vi "main.vi"() -> ()   [LabVIEW 2018]
uses:
  AutoExp/AutoExp.lvclass
  AutoExp/AutoExp.lvclass/AutoExp.ctl
  Channel/Channel.lvclass/Channel.ctl
  File interpreter/File interpreter.lvclass/File interpreter.ctl
  Channel/Channel.lvclass
  RxTx/RxTx.lvclass
  State Machine/State Machine.lvclass
  File interpreter/File interpreter.lvclass
  JSON reader/JSON reader.lvclass
  Interface/Interface.lvclass
panel:
  out "Error Out":errorcluster
  in  "Tab Control":enum32{"Acquisition", "JSON Tool"}(tab)
  out "Wait time":u16
  out "Wait time":u16
  out "Wait time":u16
  out "Wait time":u16
  out "Serial Number":u16
  out "Channel 4":bool
  out "CH4 Acquiring":bool
  out "Exp Time":dbl
  out "Temperature":i16
  out "CH4 CCD Status":string
  out "CH4 Exposures done":u8(slide) caption="Exposures done" max=1 scale=0.0..1.0
  out "CH4 Image Name":string
  out "CH4 Temp Status":string
  out "Serial Number":u16
  out "Channel 3":bool
  out "CH3 Acquiring":bool
  out "Exp Time":dbl
  out "Temperature":i16
  out "CH3 CCD Status":string
  out "CH3 Exposures done":u8(slide) caption="Exposures done" max=1 scale=0.0..1.0
  out "CH3 Image Name":string
  out "CH3 Temp Status":string
  out "Serial Number":u16
  out "Channel 2":bool
  out "CH2 Acquiring":bool
  out "Exp Time":dbl
  out "Temperature":i16
  out "CH2 CCD Status":string
  out "CH2 Exposures done":u8(slide) caption="Exposures done" max=1 scale=0.0..1.0
  out "CH2 Image Name":string
  out "CH2 Temp Status":string
  in  "Stop Application":bool
  out "Serial Number":u16
  out "Channel 1":bool
  in  "Start Acquisition":bool
  out "Acquiring":bool
  in  "Script file":path
  out "Exp Time":dbl
  out "Temperature":i16
  out "CCD Status":string
  out "Exposures done":u8(slide) max=1 scale=0.0..10.0
  out "Image Name":string
  out "Temp Status":string
  in  "Create JSON string":bool
  out "JSON string":string
  in  "AutoExp.lvclass":refnum<class "AutoExp.lvclass">
  # "Welcome to the SPARC4 Automatic Experiments Interface (AutoExp)"
  # "Channel 1"
  # "Channel 2"
  # "Channel 3"
  # "Channel 4"
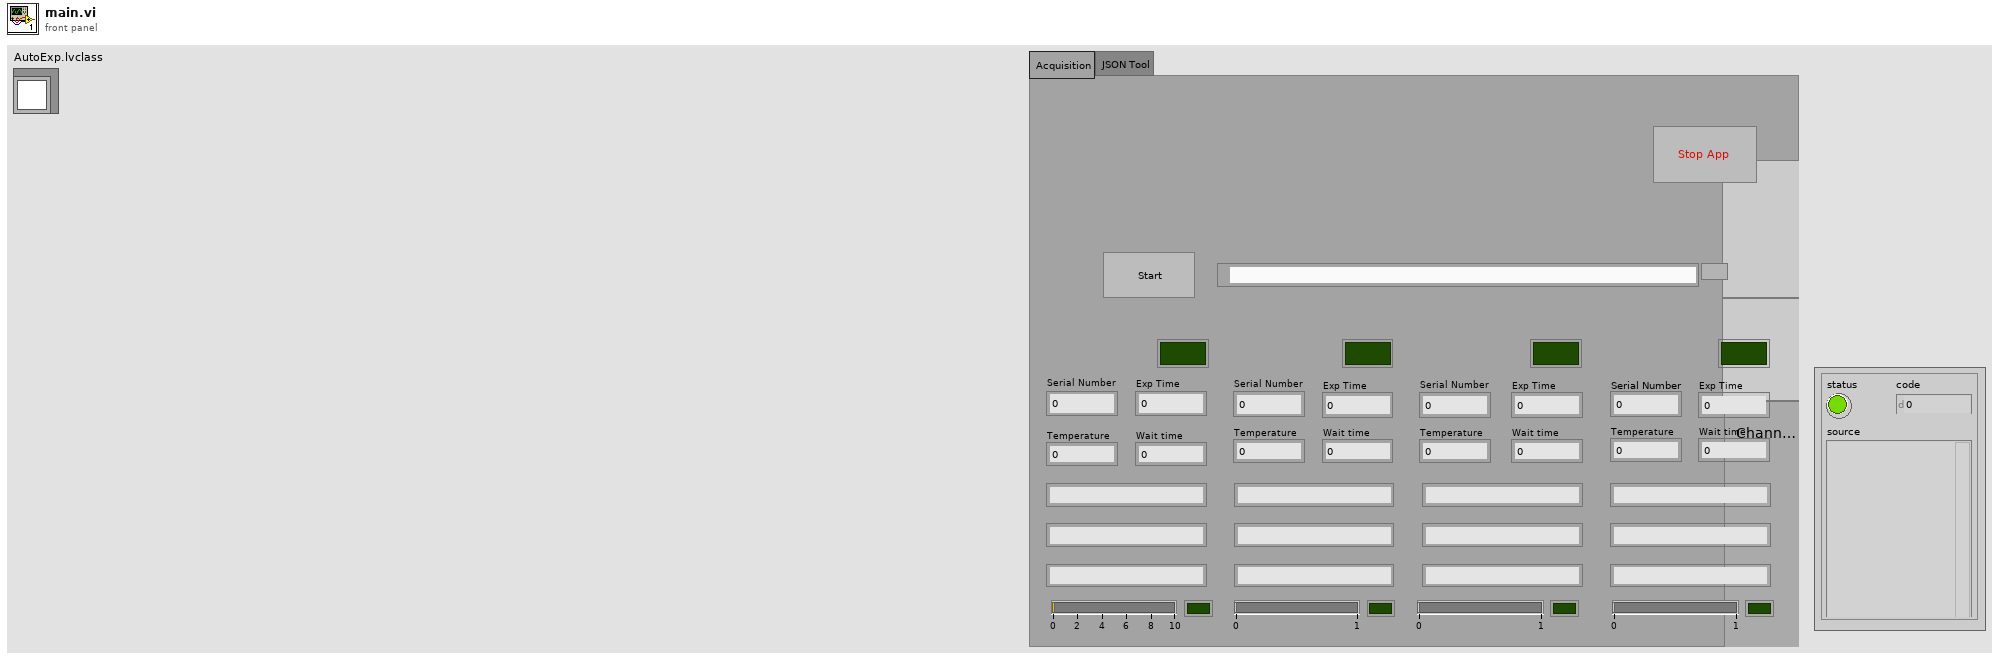
[diagram p1: front panel]
types:
  T1 = cluster{"CUBE_EXPOSURE_TIME":sgl, "CUBES_DONE":u16, "LAST_IMAGE_NAME":string, "DISK_SPACE":u16, "FRAMES_DONE":u16, "CCD_STATUS":string, "CURRENT_TEMPERATURE":i16, "TEMPERATURE_STATUS":string, "FRAME_EXPOSURE_TIME":u16, "CCD_ON_OFF":bool, "SERIAL_NUMBER":u16, "ACQUIRING":bool}
  T2 = cluster{"Exposure Time":sgl, "Pre-amp gain":u8, "Readout Rate":u8, "EM Mode":u8, "EM Gain":u16, "Binning":u16, "Initial Line":u16, "Initial Cloumn":u16, "Final Line":u16, "Final Column":u16, "Kinetic Series Length":u32, "Shutter Mode":u8, "Cooler ON/OFF":u16, "Temperature":i8, "Cubes":u32, "Trigger":u16, "Set Trigger":bool}
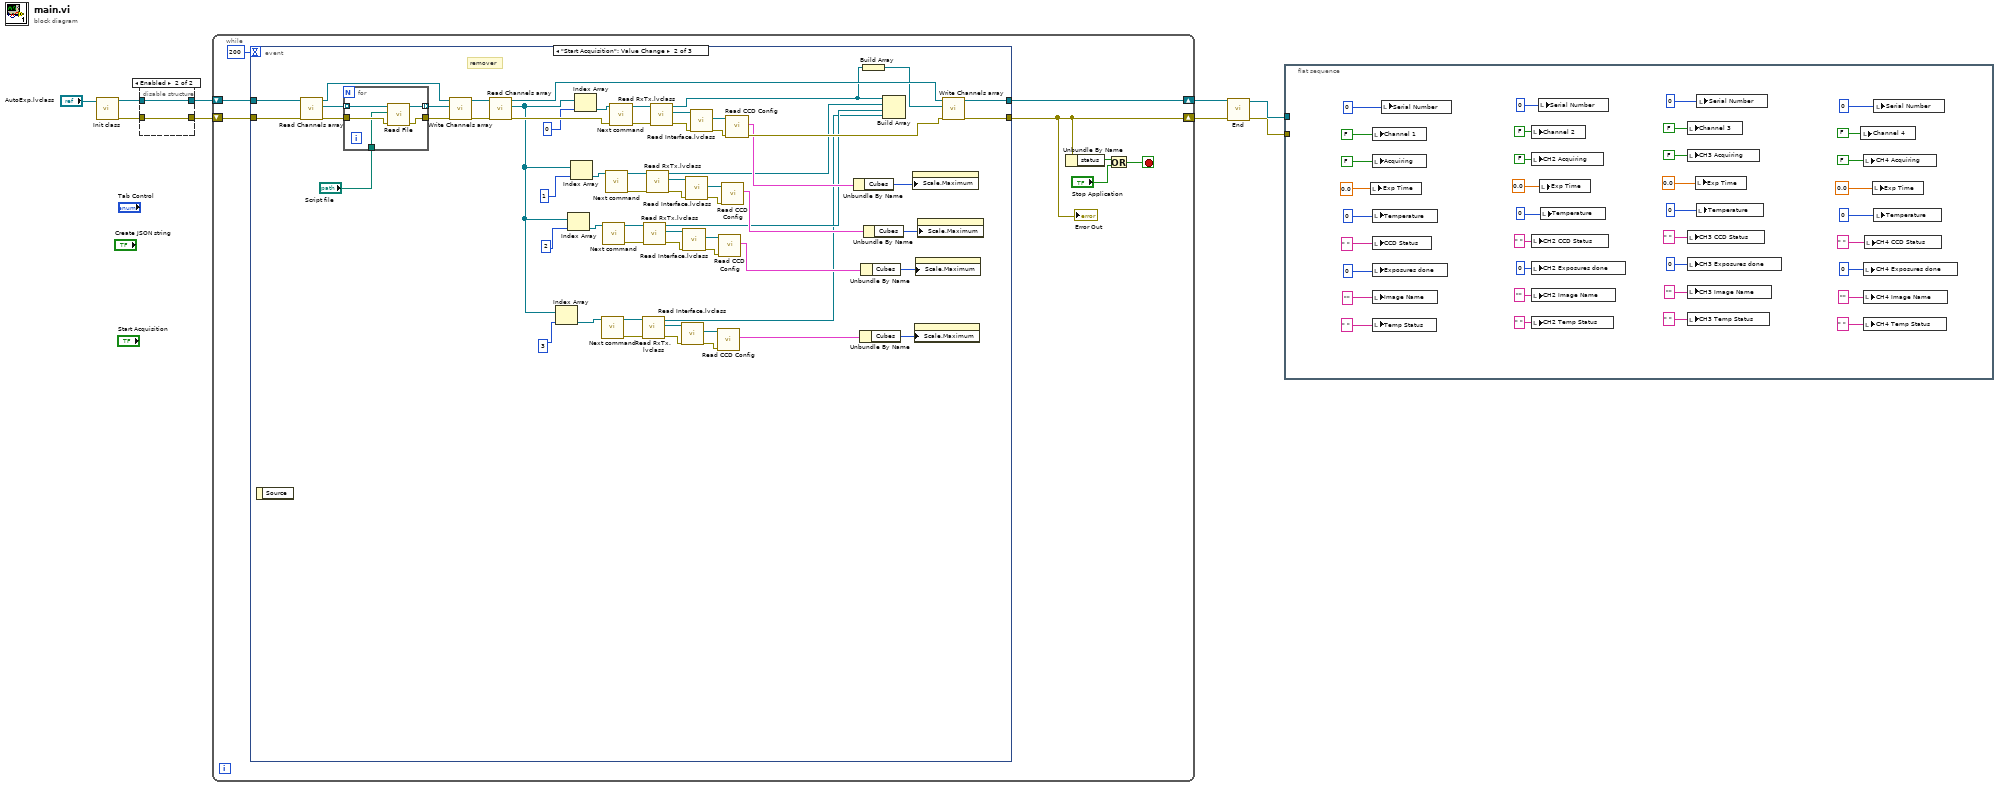
[diagram p0: block diagram]
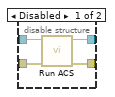
[diagram p2: hidden frame]
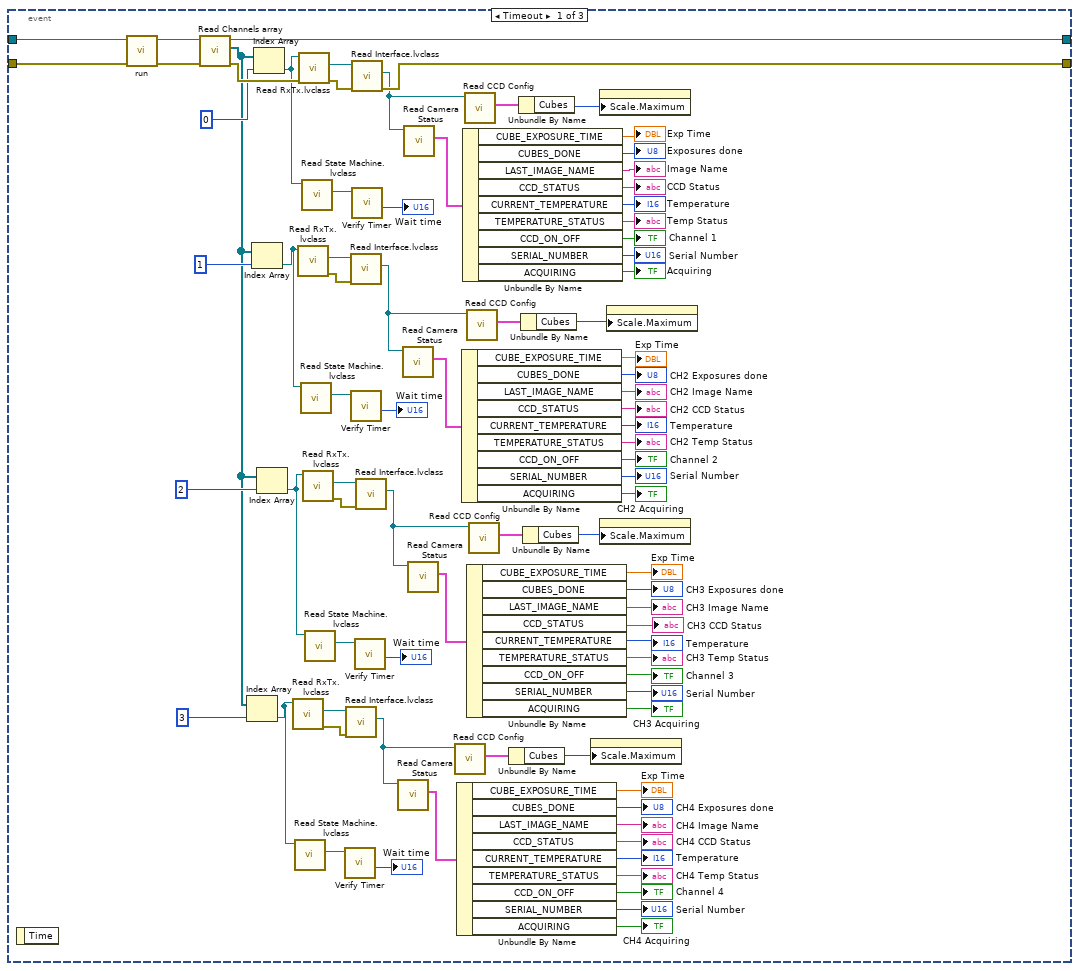
[diagram p3: hidden frame]
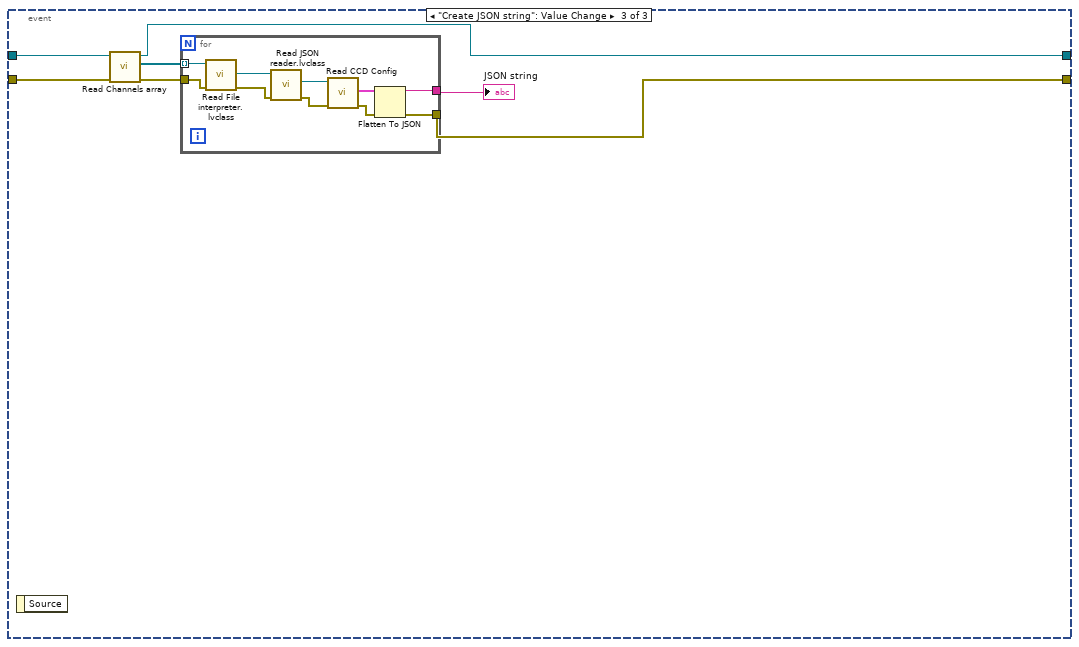
[diagram p4: hidden frame]
diagram:
  n1 = call "Init class.vi"("AutoExp in"="AutoExp.lvclass") -> ("error out"=w4:errorcluster, "AutoExp out"=w7:refnum<class "AutoExp.lvclass">)  [unwired: 9 in]
  n2 = disable-structure shown="Enabled" {
    disable-tunnel: w7 -> [w13 w15]
    disable-tunnel: [w12 w15] -> w6
    disable-tunnel: [w11 w14] -> w5
    disable-tunnel: w4 -> [w10 w14]
    frame Disabled {
      n3 = call "Run ACS.vi"("error in (no error)"=w10, "AutoExp in"=w13) -> ("error out"=w11:errorcluster, "AutoExp out"=w12:refnum<class "AutoExp.lvclass">)  [unwired: 8 in]
    }
    frame Enabled {
    }
  }
  n4 = while {
    shift-right: [w16] -> w1
    shift-left: w5 -> [w20]
    shift-right: [w21] -> w9
    shift-left: w6 -> [w22]
    stop <- w19 stop-if-true
    n5 = event shown="[1] \"Start Acquisition\": Value Change" {
      selector: _ -> [_ _ _]
      dyn-events: _ -> [_ _ _]
      timeout: 200 -> [_ _ _]
      tunnel: w22 -> [w107 w115 w180]
      tunnel: [w102 w168 w175] -> w21
      tunnel: [w101 w167 w174] -> w16
      tunnel: w20 -> [w106 w114 w179]
      event Timeout {
        n6 = event-data() -> ()  [unwired: 1 in, 1 out]
        n7 = call "run.vi"("error in (no error)"=w106, "AutoExp in"=w107) -> ("error out"=w104:errorcluster, "AutoExp out"=w105:refnum<class "AutoExp.lvclass">)  [unwired: 8 in]
        n8 = call "Read Channels array.vi"("error in (no error)"=w104, "AutoExp in"=w105) -> ("error out"=w103:errorcluster, "Channels array"=w65:refnum<class "Channel.lvclass">[], "AutoExp out"=w102:refnum<class "AutoExp.lvclass">)  [unwired: 7 in]
        n9 = Index Array(array=w65, index=3) -> (element=w41:refnum<class "Channel.lvclass">)
        n10 = Index Array(array=w65, index=1) -> (element=w47:refnum<class "Channel.lvclass">)
        n11 = Index Array(array=w65, index=0) -> (element=w51:refnum<class "Channel.lvclass">)
        n12 = Index Array(array=w65, index=2) -> (element=w44:refnum<class "Channel.lvclass">)
        n13 = call "Read RxTx.lvclass.vi"("Channel in"=w41) -> ("error out"=w63:errorcluster, "RxTx.lvclass"=w64:refnum<class "RxTx.lvclass">)  [unwired: 8 in, 1 out]
        n14 = call "Read State Machine.lvclass.vi"("Channel in"=w41) -> ("State Machine.lvclass"=w42:refnum<class "State Machine.lvclass">)  [unwired: 8 in, 2 out]
        n15 = call "Read RxTx.lvclass.vi"("Channel in"=w47) -> ("error out"=w88:errorcluster, "RxTx.lvclass"=w87:refnum<class "RxTx.lvclass">)  [unwired: 8 in, 1 out]
        n16 = call "Read RxTx.lvclass.vi"("error in (no error)"=w103, "Channel in"=w51) -> ("error out"=w99:errorcluster, "RxTx.lvclass"=w100:refnum<class "RxTx.lvclass">)  [unwired: 7 in, 1 out]
        n17 = call "Read State Machine.lvclass.vi"("Channel in"=w47) -> ("State Machine.lvclass"=w48:refnum<class "State Machine.lvclass">)  [unwired: 8 in, 2 out]
        n18 = call "Read State Machine.lvclass.vi"("Channel in"=w51) -> ("State Machine.lvclass"=w50:refnum<class "State Machine.lvclass">)  [unwired: 8 in, 2 out]
        n19 = call "Read RxTx.lvclass.vi"("Channel in"=w44) -> ("error out"=w74:errorcluster, "RxTx.lvclass"=w75:refnum<class "RxTx.lvclass">)  [unwired: 8 in, 1 out]
        n20 = call "Read State Machine.lvclass.vi"("Channel in"=w44) -> ("State Machine.lvclass"=w45:refnum<class "State Machine.lvclass">)  [unwired: 8 in, 2 out]
        n21 = call "Verify Timer.vi"("State Machine in"=w42) -> ("elapsed time"=→"Wait time":u16)  [unwired: 7 in, 3 out]
        n22 = call "Read Interface.lvclass.vi"("error in (no error)"=w63, "RxTx in"=w64) -> ("Interface.lvclass"=w25:refnum<class "Interface.lvclass">)  [unwired: 7 in, 2 out]
        n23 = call "Read Interface.lvclass.vi"("error in (no error)"=w88, "RxTx in"=w87) -> ("Interface.lvclass"=w31:refnum<class "Interface.lvclass">)  [unwired: 7 in, 2 out]
        n24 = call "Verify Timer.vi"("State Machine in"=w48) -> ("elapsed time"=→"Wait time":u16)  [unwired: 7 in, 3 out]
        n25 = call "Read Interface.lvclass.vi"("error in (no error)"=w99, "RxTx in"=w100) -> ("error out"=w101:errorcluster, "Interface.lvclass"=w35:refnum<class "Interface.lvclass">)  [unwired: 7 in, 1 out]
        n26 = call "Verify Timer.vi"("State Machine in"=w50) -> ("elapsed time"=→"Wait time":u16)  [unwired: 7 in, 3 out]
        n27 = call "Verify Timer.vi"("State Machine in"=w45) -> ("elapsed time"=→"Wait time":u16)  [unwired: 7 in, 3 out]
        n28 = call "Read Interface.lvclass.vi"("error in (no error)"=w74, "RxTx in"=w75) -> ("Interface.lvclass"=w28:refnum<class "Interface.lvclass">)  [unwired: 7 in, 2 out]
        n29 = call "Read Camera Status.vi"("Interface in"=w25) -> ("Camera Status"=w57:T1)  [unwired: 8 in, 2 out]
        n30 = call "Read Camera Status.vi"("Interface in"=w31) -> ("Camera Status"=w89:T1)  [unwired: 8 in, 2 out]
        n31 = call "Read Camera Status.vi"("Interface in"=w35) -> ("Camera Status"=w98:T1)  [unwired: 8 in, 2 out]
        n32 = call "Read Camera Status.vi"("Interface in"=w28) -> ("Camera Status"=w73:T1)  [unwired: 8 in, 2 out]
        n33 = call "Read CCD Config.vi"("Interface in"=w25) -> ("CCD Config"=w26:T2)  [unwired: 8 in, 2 out]
        n34 = Unbundle By Name(w57) -> ("CUBE_EXPOSURE_TIME"=→"Exp Time":sgl, "CUBES_DONE"=→"CH4 Exposures done":u16, "LAST_IMAGE_NAME"=→"CH4 Image Name":string, "CCD_STATUS"=→"CH4 CCD Status":string, "CURRENT_TEMPERATURE"=→"Temperature":i16, "TEMPERATURE_STATUS"=→"CH4 Temp Status":string, "CCD_ON_OFF"=→"Channel 4":bool, "SERIAL_NUMBER"=→"Serial Number":u16, "ACQUIRING"=→"CH4 Acquiring":bool)
        n35 = Unbundle By Name(w89) -> ("CUBE_EXPOSURE_TIME"=→"Exp Time":sgl, "CUBES_DONE"=→"CH2 Exposures done":u16, "LAST_IMAGE_NAME"=→"CH2 Image Name":string, "CCD_STATUS"=→"CH2 CCD Status":string, "CURRENT_TEMPERATURE"=→"Temperature":i16, "TEMPERATURE_STATUS"=→"CH2 Temp Status":string, "CCD_ON_OFF"=→"Channel 2":bool, "SERIAL_NUMBER"=→"Serial Number":u16, "ACQUIRING"=→"CH2 Acquiring":bool)
        n36 = Unbundle By Name(w98) -> ("CUBE_EXPOSURE_TIME"=→"Exp Time":sgl, "CUBES_DONE"=→"Exposures done":u16, "LAST_IMAGE_NAME"=→"Image Name":string, "CCD_STATUS"=→"CCD Status":string, "CURRENT_TEMPERATURE"=→"Temperature":i16, "TEMPERATURE_STATUS"=→"Temp Status":string, "CCD_ON_OFF"=→"Channel 1":bool, "SERIAL_NUMBER"=→"Serial Number":u16, "ACQUIRING"=→"Acquiring":bool)
        n37 = call "Read CCD Config.vi"("Interface in"=w35) -> ("CCD Config"=w34:T2)  [unwired: 8 in, 2 out]
        n38 = call "Read CCD Config.vi"("Interface in"=w31) -> ("CCD Config"=w32:T2)  [unwired: 8 in, 2 out]
        n39 = Unbundle By Name(w73) -> ("CUBE_EXPOSURE_TIME"=→"Exp Time":sgl, "CUBES_DONE"=→"CH3 Exposures done":u16, "LAST_IMAGE_NAME"=→"CH3 Image Name":string, "CCD_STATUS"=→"CH3 CCD Status":string, "CURRENT_TEMPERATURE"=→"Temperature":i16, "TEMPERATURE_STATUS"=→"CH3 Temp Status":string, "CCD_ON_OFF"=→"Channel 3":bool, "SERIAL_NUMBER"=→"Serial Number":u16, "ACQUIRING"=→"CH3 Acquiring":bool)
        n40 = call "Read CCD Config.vi"("Interface in"=w28) -> ("CCD Config"=w29:T2)  [unwired: 8 in, 2 out]
        n41 = Unbundle By Name(w26) -> ("Cubes"=w24:u32)
        n42 = Unbundle By Name(w34) -> ("Cubes"=w33:u32)
        n43 = Unbundle By Name(w32) -> ("Cubes"=w30:u32)
        n44 = Unbundle By Name(w29) -> ("Cubes"=w27:u32)
        n45 = property on="CH4 Exposures done" class="Slide (strict)"("Scale.Maximum"=w24) -> ()  [unwired: 2 in, 2 out]
        n46 = property on="Exposures done" class="Slide (strict)"("Scale.Maximum"=w33) -> ()  [unwired: 2 in, 2 out]
        n47 = property on="CH3 Exposures done" class="Slide (strict)"("Scale.Maximum"=w27) -> ()  [unwired: 2 in, 2 out]
        n48 = property on="CH2 Exposures done" class="Slide (strict)"("Scale.Maximum"=w30) -> ()  [unwired: 2 in, 2 out]
      }
      event "Start Acquisition": Value Change {
        # "remover"
        n49 = event-data() -> ()  [unwired: 1 in, 1 out]
        n50 = call "Read Channels array.vi"("error in (no error)"=w114, "AutoExp in"=w115) -> ("error out"=w118:errorcluster, "Channels array"=w120:refnum<class "Channel.lvclass">[], "AutoExp out"=w116:refnum<class "AutoExp.lvclass">)  [unwired: 7 in]
        n51 = for {
          tunnel: w120 -> [w173] mode=indexing
          tunnel: [w172] -> w119 mode=indexing
          tunnel: w118 -> [w171]
          tunnel: [w170] -> w117
          tunnel: "Script file" -> [w169]
          n52 = call "Read File.vi"("error in (no error)"=w171, "file path (use dialog)"=w169, "Channel in"=w173) -> ("error out"=w170:errorcluster, "Channel out"=w172:refnum<class "Channel.lvclass">)  [unwired: 7 in]
        }
        n53 = call "Write Channels array.vi"("error in (no error)"=w117, "Channels array"=w119, "AutoExp in"=w116) -> ("error out"=w112:errorcluster, "AutoExp out"=w113:refnum<class "AutoExp.lvclass">)  [unwired: 7 in]
        n54 = call "Read Channels array.vi"("error in (no error)"=w112, "AutoExp in"=w113) -> ("error out"=w165:errorcluster, "Channels array"=w110:refnum<class "Channel.lvclass">[], "AutoExp out"=w166:refnum<class "AutoExp.lvclass">)  [unwired: 7 in]
        n55 = Index Array(array=w110, index=3) -> (element=w131:refnum<class "Channel.lvclass">)
        n56 = Index Array(array=w110, index=2) -> (element=w142:refnum<class "Channel.lvclass">)
        n57 = Index Array(array=w110, index=1) -> (element=w148:refnum<class "Channel.lvclass">)
        n58 = Index Array(array=w110, index=0) -> (element=w156:refnum<class "Channel.lvclass">)
        n59 = call "Next command.vi"("Channel in"=w131) -> ("error out"=w133:errorcluster, "Channel out"=w130:refnum<class "Channel.lvclass">)  [unwired: 9 in]
        n60 = call "Next command.vi"("Channel in"=w142) -> ("error out"=w140:errorcluster, "Channel out"=w143:refnum<class "Channel.lvclass">)  [unwired: 9 in]
        n61 = call "Next command.vi"("Channel in"=w148) -> ("error out"=w150:errorcluster, "Channel out"=w147:refnum<class "Channel.lvclass">)  [unwired: 9 in]
        n62 = call "Next command.vi"("error in (no error)"=w165, "Channel in"=w156) -> ("error out"=w162:errorcluster, "Channel out"=w163:refnum<class "Channel.lvclass">)  [unwired: 8 in]
        n63 = call "Read RxTx.lvclass.vi"("error in (no error)"=w133, "Channel in"=w130) -> ("error out"=w134:errorcluster, "RxTx.lvclass"=w129:refnum<class "RxTx.lvclass">, "Channel out"=w122:refnum<class "Channel.lvclass">)  [unwired: 7 in]
        n64 = call "Read RxTx.lvclass.vi"("error in (no error)"=w140, "Channel in"=w143) -> ("error out"=w139:errorcluster, "RxTx.lvclass"=w144:refnum<class "RxTx.lvclass">, "Channel out"=w123:refnum<class "Channel.lvclass">)  [unwired: 7 in]
        n65 = call "Read RxTx.lvclass.vi"("error in (no error)"=w150, "Channel in"=w147) -> ("error out"=w151:errorcluster, "RxTx.lvclass"=w146:refnum<class "RxTx.lvclass">, "Channel out"=w124:refnum<class "Channel.lvclass">)  [unwired: 7 in]
        n66 = call "Read RxTx.lvclass.vi"("error in (no error)"=w162, "Channel in"=w163) -> ("error out"=w160:errorcluster, "RxTx.lvclass"=w161:refnum<class "RxTx.lvclass">, "Channel out"=w109:refnum<class "Channel.lvclass">)  [unwired: 7 in]
        n67 = call "Read Interface.lvclass.vi"("error in (no error)"=w134, "RxTx in"=w129) -> ("error out"=w136:errorcluster, "Interface.lvclass"=w135:refnum<class "Interface.lvclass">)  [unwired: 7 in, 1 out]
        n68 = call "Read Interface.lvclass.vi"("error in (no error)"=w139, "RxTx in"=w144) -> ("error out"=w137:errorcluster, "Interface.lvclass"=w138:refnum<class "Interface.lvclass">)  [unwired: 7 in, 1 out]
        n69 = call "Read Interface.lvclass.vi"("error in (no error)"=w151, "RxTx in"=w146) -> ("error out"=w153:errorcluster, "Interface.lvclass"=w152:refnum<class "Interface.lvclass">)  [unwired: 7 in, 1 out]
        n70 = call "Read Interface.lvclass.vi"("error in (no error)"=w160, "RxTx in"=w161) -> ("error out"=w158:errorcluster, "Interface.lvclass"=w159:refnum<class "Interface.lvclass">)  [unwired: 7 in, 1 out]
        n71 = call "Read CCD Config.vi"("error in (no error)"=w136, "Interface in"=w135) -> ("CCD Config"=w128:T2)  [unwired: 7 in, 2 out]
        n72 = call "Read CCD Config.vi"("error in (no error)"=w137, "Interface in"=w138) -> ("CCD Config"=w126:T2)  [unwired: 7 in, 2 out]
        n73 = call "Read CCD Config.vi"("error in (no error)"=w153, "Interface in"=w152) -> ("CCD Config"=w154:T2)  [unwired: 7 in, 2 out]
        n74 = call "Read CCD Config.vi"("error in (no error)"=w158, "Interface in"=w159) -> ("error out"=w164:errorcluster, "CCD Config"=w157:T2)  [unwired: 7 in, 1 out]
        n75 = Unbundle By Name(w157) -> ("Cubes"=w111:u32)
        n76 = Unbundle By Name(w128) -> ("Cubes"=w127:u32)
        n77 = Unbundle By Name(w126) -> ("Cubes"=w125:u32)
        n78 = Build Array(w109) -> (w108:refnum<class "Channel.lvclass">[])
        n79 = Unbundle By Name(w154) -> ("Cubes"=w145:u32)
        n80 = Build Array(w109, w124, w123, w122) -> ()  [unwired: 1 out]
        n81 = property on="Exposures done" class="Slide (strict)"("Scale.Maximum"=w111) -> ()  [unwired: 2 in, 2 out]
        n82 = property on="CH4 Exposures done" class="Slide (strict)"("Scale.Maximum"=w127) -> ()  [unwired: 2 in, 2 out]
        n83 = property on="CH3 Exposures done" class="Slide (strict)"("Scale.Maximum"=w125) -> ()  [unwired: 2 in, 2 out]
        n84 = property on="CH2 Exposures done" class="Slide (strict)"("Scale.Maximum"=w145) -> ()  [unwired: 2 in, 2 out]
        n85 = call "Write Channels array.vi"("error in (no error)"=w164, "Channels array"=w108, "AutoExp in"=w166) -> ("error out"=w167:errorcluster, "AutoExp out"=w168:refnum<class "AutoExp.lvclass">)  [unwired: 7 in]
      }
      event "Create JSON string": Value Change {
        n86 = event-data() -> ()  [unwired: 1 in, 1 out]
        n87 = call "Read Channels array.vi"("error in (no error)"=w179, "AutoExp in"=w180) -> ("error out"=w177:errorcluster, "Channels array"=w178:refnum<class "Channel.lvclass">[], "AutoExp out"=w175:refnum<class "AutoExp.lvclass">)  [unwired: 7 in]
        n88 = for {
          tunnel: w178 -> [w190] mode=indexing
          tunnel: w177 -> [w187]
          tunnel: [w182] -> w176
          tunnel: [w181] -> w174
          n89 = call "Read File interpreter.lvclass.vi"("error in (no error)"=w187, "Channel in"=w190) -> ("error out"=w188:errorcluster, "File interpreter.lvclass"=w189:refnum<class "File interpreter.lvclass">)  [unwired: 7 in, 1 out]
          n90 = call "Read JSON reader.lvclass.vi"("error in (no error)"=w188, "File interpreter in"=w189) -> ("error out"=w185:errorcluster, "JSON reader.lvclass"=w186:refnum<class "JSON reader.lvclass">)  [unwired: 7 in, 1 out]
          n91 = call "Read CCD Config.vi"("error in (no error)"=w185, "JSON reader in"=w186) -> ("error out"=w184:errorcluster, "CCD Config"=w183:T2)  [unwired: 7 in, 1 out]
          n92 = Flatten To JSON(anything=w183, error in (no error)=w184) -> (JSON string=w182:string, 11:w181:errorcluster)  [unwired: 1 in]
        }
        "JSON string" <- w176
      }
    }
    "Error Out" <- w16
    n93 = Unbundle By Name(w16) -> ("status"=w17:bool)
    n94 = Or(x=w17, y="Stop Application") -> (x .or. y?=w19:bool)
  }
  n95 = call "End.vi"("error in (no error)"=w1, "AutoExp in"=w9) -> ("error out"=w2:errorcluster, "AutoExp out"=w3:refnum<class "AutoExp.lvclass">)  [unwired: 8 in]
  n96 = flat-sequence {
    tunnel: w3 -> [_]
    tunnel: w2 -> [_]
    frame #0 {
      n97 = local write "Exp Time"(0.0 ("CH2 ExpTime")) -> ()
      n98 = local write "Channel 1"(FALSE ("Channel 2")) -> ()
      n99 = local write "Acquiring"(FALSE ("CH2 Acquiring")) -> ()
      n100 = local write "Temperature"(i16 0 ("CH2 Temperature")) -> ()
      n101 = local write "CCD Status"(" " ("CH2 CCD Status")) -> ()
      n102 = local write "Exposures done"(u8 0 ("CH2 Exposures done")) -> ()
      n103 = local write "Image Name"("" ("CH2 Image Name")) -> ()
      n104 = local write "Temp Status"(" " ("CH2 Temp Status")) -> ()
      n105 = local write "Serial Number"(u16 0 ("CH Serial Number")) -> ()
      n106 = local write "Channel 2"(FALSE ("Channel 2")) -> ()
      n107 = local write "CH2 Acquiring"(FALSE ("CH2 Acquiring")) -> ()
      n108 = local write "CH2 CCD Status"(" " ("CH2 CCD Status")) -> ()
      n109 = local write "CH2 Exposures done"(u8 0 ("CH2 Exposures done")) -> ()
      n110 = local write "CH2 Image Name"("" ("CH2 Image Name")) -> ()
      n111 = local write "CH2 Temp Status"(" " ("CH2 Temp Status")) -> ()
      n112 = local write "Serial Number"(u16 0 ("CH Serial Number")) -> ()
      n113 = local write "Exp Time"(0.0 ("CH2 ExpTime")) -> ()
      n114 = local write "Temperature"(i16 0 ("CH2 Temperature")) -> ()
      n115 = local write "Channel 3"(FALSE ("Channel 2")) -> ()
      n116 = local write "CH3 Acquiring"(FALSE ("CH2 Acquiring")) -> ()
      n117 = local write "CH3 CCD Status"(" " ("CH2 CCD Status")) -> ()
      n118 = local write "CH3 Exposures done"(u8 0 ("CH2 Exposures done")) -> ()
      n119 = local write "CH3 Image Name"("" ("CH2 Image Name")) -> ()
      n120 = local write "CH3 Temp Status"(" " ("CH2 Temp Status")) -> ()
      n121 = local write "Exp Time"(0.0 ("CH2 ExpTime")) -> ()
      n122 = local write "Temperature"(i16 0 ("CH2 Temperature")) -> ()
      n123 = local write "Serial Number"(u16 0 ("CH Serial Number")) -> ()
      n124 = local write "Channel 4"(FALSE ("Channel 2")) -> ()
      n125 = local write "CH4 Acquiring"(FALSE ("CH2 Acquiring")) -> ()
      n126 = local write "CH4 Exposures done"(u8 0 ("CH2 Exposures done")) -> ()
      n127 = local write "CH4 Image Name"("" ("CH2 Image Name")) -> ()
      n128 = local write "CH4 Temp Status"(" " ("CH2 Temp Status")) -> ()
      n129 = local write "CH4 CCD Status"(" " ("CH2 CCD Status")) -> ()
      n130 = local write "Exp Time"(0.0 ("CH2 ExpTime")) -> ()
      n131 = local write "Serial Number"(u16 0 ("CH Serial Number")) -> ()
      n132 = local write "Temperature"(i16 0 ("CH2 Temperature")) -> ()
    }
  }
